vi "cRIO Test Demo.vi"() -> ()   [LabVIEW 2011]
panel:
  out "MAC Address 2":string
  out "Personality 2":string
  out "Personality":string
  in  "4 slot cRIO":string="[GENERAL]\nMACAddress=\"ABCD1234EFGH;\"\nPrimary MAC=\"ABCD1234EFGH\""
  in  "8 Slot cRIO":string="[abcd9876efgh]\nmode=\"TCPIP\"\nIP_Address=\"192.168.0.3\"\nSubnet_mask=\"255.255.255.0\""
  out "File Text":string
  in  "4 ?":bool
  out "MAC Address":string
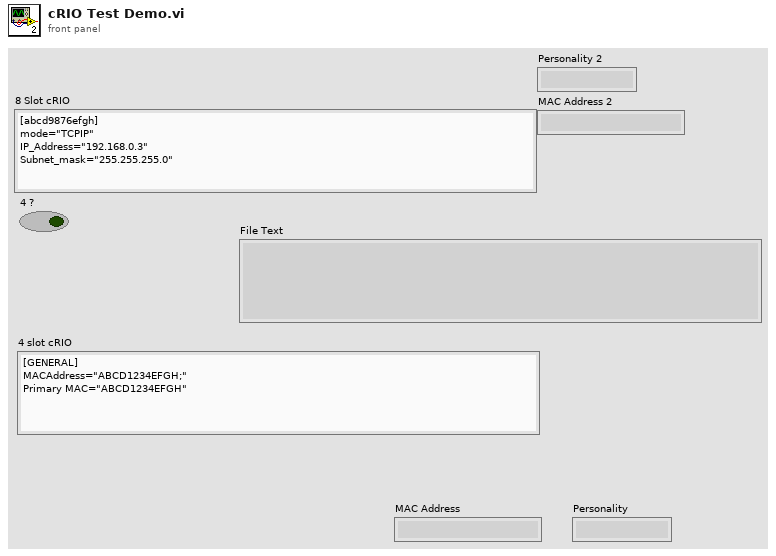
[diagram p1: front panel]
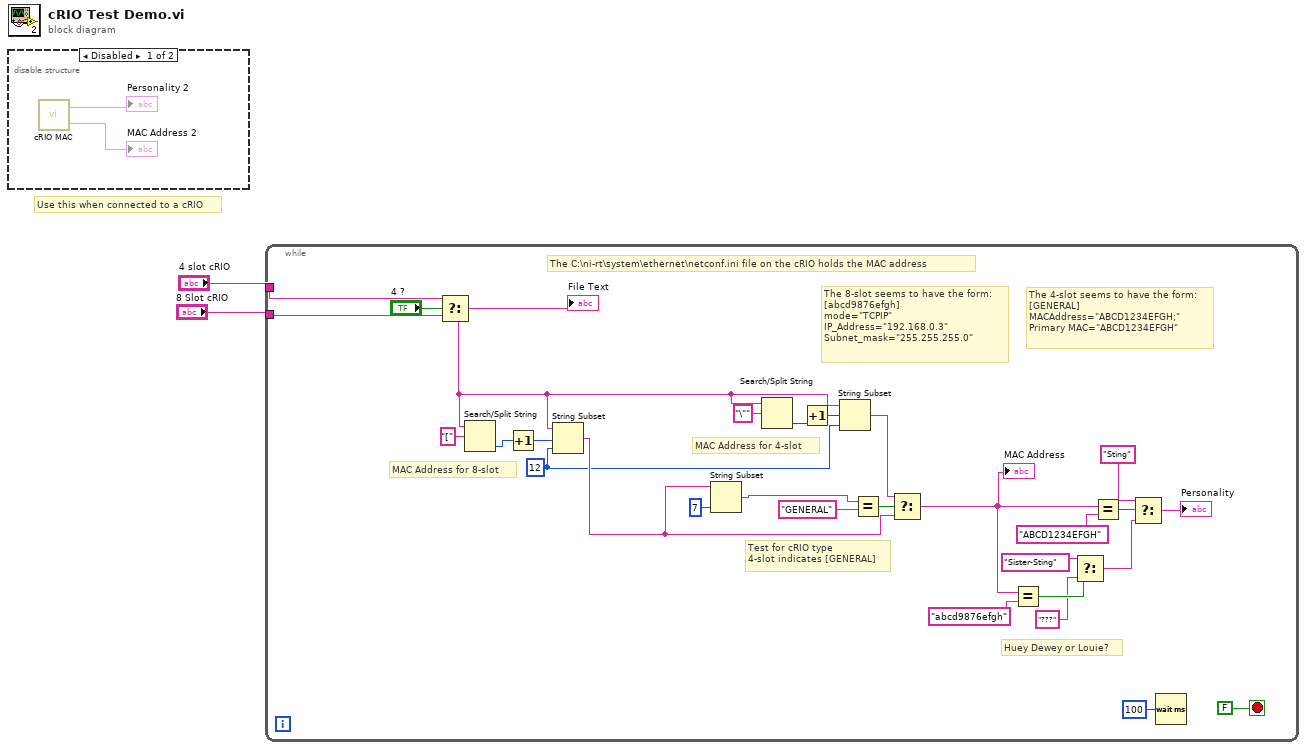
[diagram p0: block diagram]
diagram:
  # "Use this when connected to a cRIO"
  n1 = disable-structure shown="Disabled" {
    frame Disabled {
      n2 = call "cRIO MAC.vi"() -> ("MAC Address"=→"MAC Address 2":string, "Personality"=→"Personality 2":string)  [unwired: 2 in]
    }
    frame Enabled {
    }
  }
  n3 = while {
    tunnel: "4 slot cRIO" -> [w24]
    tunnel: "8 Slot cRIO" -> [w23]
    stop <- FALSE stop-if-true
    w17 = 12 ("length (rest)")
    # "Huey Dewey or Louie?"
    # "MAC Address for 4-slot"
    # "MAC Address for 8-slot"
    # "The 4-slot seems to have the form:\n[GENERAL]\nMACAddress=\"ABCD1234EFGH;\"\nPrimary MAC=\"ABCD1234EFGH\""
    # "The 8-slot seems to have the form:\n[abcd9876efgh]\nmode=\"TCPIP\"\nIP_Address=\"192.168.0.3\"\nSubnet_mask=\"255.255.255.0\""
    # "The C:\\ni-rt\\system\\ethernet\\netconf.ini file on the cRIO holds the MAC address"
    # "Test for cRIO type\n4-slot indicates [GENERAL]"
    n4 = Select(t=w24, s="4 ?", f=w23) -> (s? t:f=w20:string)
    "File Text" <- w20
    n5 = Search/Split String(string=w20, search string/char (-)="[") -> (offset of match=w32:i32)  [unwired: 1 in, 2 out]
    n6 = Increment(x=w32) -> (x+1=w33:i32)
    n7 = String Subset(string=w20, offset (0)=w33, length (rest)=w17) -> (substring=w22:string)
    n8 = String Subset(string=w22, length (rest)=7 ("length (rest)")) -> (substring=w28:string)  [unwired: 1 in]
    n9 = Search/Split String(string=w20, search string/char (-)="\"") -> (offset of match=w21:i32)  [unwired: 1 in, 2 out]
    n10 = Increment(x=w21) -> (x+1=w18:i32)
    n11 = String Subset(string=w20, offset (0)=w18, length (rest)=w17) -> (substring=w19:string)
    n12 = Equal?(x=w28, y="GENERAL") -> (x = y?=w26:bool)
    n13 = Select(t=w19, s=w26, f=w22) -> (s? t:f=w10:string)
    "MAC Address" <- w10
    n14 = Equal?(x=w10, y="abcd9876efgh") -> (x = y?=w9:bool)
    n15 = Select(t="Sister-Sting", s=w9, f="???") -> (s? t:f=w8:string)
    n16 = Equal?(x=w10, y="ABCD1234EFGH") -> (x = y?=w13:bool)
    n17 = Select(t="Sting", s=w13, f=w8) -> (s? t:f=→"Personality":string)
    n18 = Wait (ms)(milliseconds to wait=u32 100) -> ()  [unwired: 1 out]
  }
